vi "3_PatchCore_Report(Dataset).vi"(0 "NNFE PatchCore Paths":T1={"NNFE_Paths"={"CFG"=path "D:/PatchCore/__24_12_11__22_07_40/wrn_50_2_timm_NNFE__24_12_11__22_07_40.cfg", "BIN"=path "D:/PatchCore/__24_12_11__22_07_40/wrn_50_2_timm_NNFE__24_12_11__22_07_40.bin"}, "PatchCore_Paths"={"CFG"=path "D:/PatchCore/__24_12_11__22_07_40/wrn_50_2_timm_Patchcore__24_12_11__22_07_40.cfg", "BIN"=path "D:/PatchCore/__24_12_11__22_07_40/wrn_50_2_timm_MemBank__PS3_RP296_SR0.1_Size16.4k__24_12_11__22_07_40.bin"}}, 1 "NNFE_Custom_CFG":T11={"Input3D_Custom_Dims"={"C"=3, "H"=224, "W"=224}, "mBatch"=1}, 2 "Feature_Scorer_Params":T6={"Nearest_Neihbours"=1, "Calculate Anomaly Map"=TRUE, "Gaussian_Blur"={"Kernel_Size"=33, "sigma"=4.0}}, 3 "Report_Image_Dims":cluster{"X Resolution":i32, "Y Resolution":i32}={"X Resolution"=224, "Y Resolution"=224}, 7 "Eval_Stats_File_Path":path=path "D:/PatchCore/__24_12_11__22_07_40/PatchCore_Eval_Stats__24_12_11__22_13_40.cfg", 11 "Device_Config.":T3={"Device"=enum."GPU", "GPU Id"=0}, 12 "Image_Dataset_Folder_Path":path=path "D:/MVTec/bottle/test", 13 "Ground_Truth_Folder_Path":path=path "D:/MVTec/bottle/ground_truth", 14 "Dest. Path":path=path "D:/MVTec_Report/bottle") -> (6 "dt_Predict":dbl=0.010424548192794788 format="%#_4p")   [LabVIEW 2020]
uses:
  PatchCore_AddOn/API/Controls/NNPC_Init_Custom_NN_CFG.ctl
  <vilib>/Ngene/Deep Learning Toolkit/Toolkit/NN_Data/API/NN_Dims(C,H,W).ctl
  PatchCore_AddOn/API/Controls/Heatmap_Config.ctl
  PatchCore_AddOn/API/Controls/ColorMap.ctl
  PatchCore_AddOn/API/Controls/MinMax.ctl
  PatchCore_AddOn/API/Controls/Feature_Scorer_Params.ctl
  PatchCore_AddOn/API/Controls/Gaussian_Blur.ctl
  PatchCore_AddOn/API/Controls/NNPC_Device.ctl
  <vilib>/Ngene/Deep Learning Toolkit/Toolkit/NN_Network/Controls/NN_Device.ctl
  PatchCore_AddOn/API/Controls/NNPC_Trained_Model_Paths.ctl
  PatchCore_AddOn/API/Controls/NN_Paths.ctl
  subVIs/Dataset_Reader/Controls/ImRead_PreProcessing_Options.ctl
  PatchCore_AddOn/Low_Level/Controls/Normalization_Type.ctl
  <vilib>/Analysis/baseanly.llb/Mean (DBL).vi
  PatchCore_AddOn/API/NNPC_Predict/NNPC_Predict(Single).vi
  PatchCore_AddOn/PatchCore_AddOn.lvlib
  <vilib>/Analysis/NI_AALBase.lvlib
  <vilib>/Ngene/Deep Learning Toolkit/Toolkit/Deep_Learning_Toolkit_by_Ngene.lvlib
panel:
  out "Anomaly Detection Results":T5(plugin-control)
  out "Actual_Pixel_Threshold":sgl=25.5661
  out "Total":i32=83
  out "Progress":i32=82
  in  "Heatmap_Config":T8={"ColorMap_Type"=enum."Jet", "Alpha"=0.4, "Heatmap Range"={"Min"=-1.0, "Max"=-1.0}} {"Heatmap Range"."Min" format="%#_5g"}
  out "dT_ImRead":dbl=0.022437069879479934 format="%#_4p"
  in  "Pixel_Thrshld(Custom)":sgl=-1.0 format="%_5g"
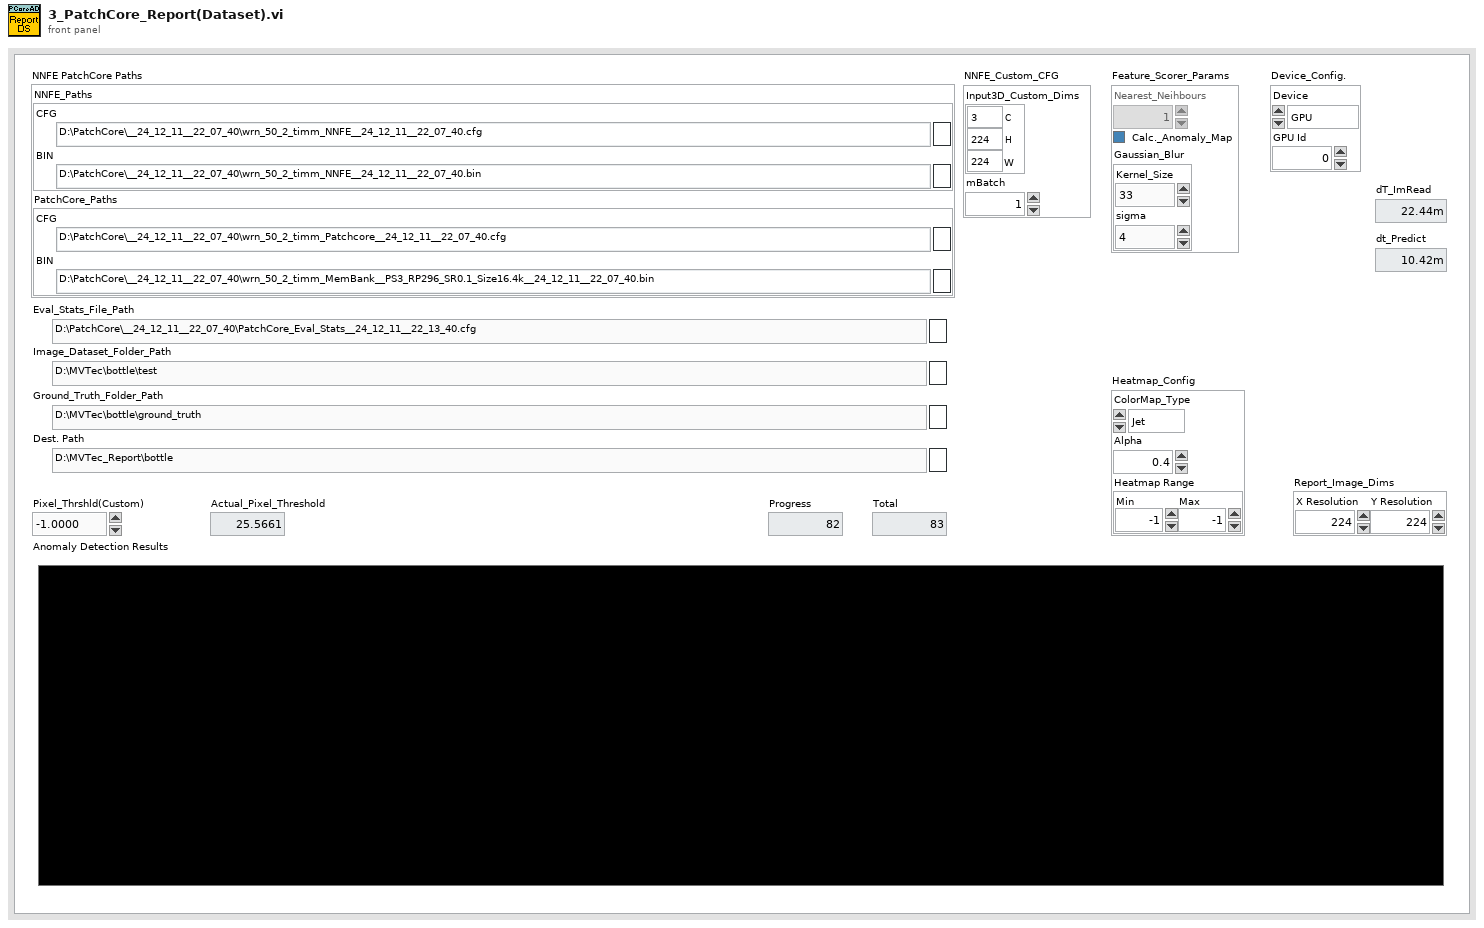
[diagram p1: front panel]
types:
  T1 = typedef "PatchCore_AddOn.lvlib/NNPC_Trained_Model_Paths.ctl" = cluster{"NNFE_Paths":T2, "PatchCore_Paths":T2}
  T2 = typedef "PatchCore_AddOn.lvlib/NN_Paths.ctl" = cluster{"CFG":path, "BIN":path}
  T3 = typedef "PatchCore_AddOn.lvlib/NNPC_Device.ctl" = cluster{"Device":T4, "GPU Id":i32}
  T4 = typedef "Deep_Learning_Toolkit_by_Ngene.lvlib/NN_Device.ctl" = enum16{"CPU", "GPU"}
  T5 = typedef "IMAQ Image.ctl" = refnum<image>
  T6 = typedef "PatchCore_AddOn.lvlib/Feature_Scorer_Params.ctl" = cluster{"Nearest_Neihbours":i32, "Calculate Anomaly Map":bool, "Gaussian_Blur":T7}
  T7 = typedef "PatchCore_AddOn.lvlib/Gaussian_Blur.ctl" = cluster{"Kernel_Size":i32, "sigma":sgl}
  T8 = typedef "PatchCore_AddOn.lvlib/Heatmap_Config.ctl" = cluster{"ColorMap_Type":T9, "Alpha":sgl, "Heatmap Range":T10}
  T9 = typedef "PatchCore_AddOn.lvlib/ColorMap.ctl" = enum16{"Jet", "Perula", "Inferno", "Plasma", "Viridis"}
  T10 = typedef "PatchCore_AddOn.lvlib/MinMax.ctl" = cluster{"Min":sgl, "Max":sgl}
  T11 = typedef "PatchCore_AddOn.lvlib/NNPC_Init_Custom_NN_CFG.ctl" = cluster{"Input3D_Custom_Dims":T12, "mBatch":i32}
  T12 = typedef "Deep_Learning_Toolkit_by_Ngene.lvlib/NN_Dims(C,H,W).ctl" = cluster{"C":i32, "H":i32, "W":i32}
  T13 = typedef "PatchCore_AddOn.lvlib/NNPC_Instance.ctl" = cluster{"Dataset_Stats":T14, "NN":T16, "Device_Config.":T3, "PatchCore_Init_CFG":T31, "Coreset Params":T33, "MemBank_Data":T35}
  T14 = typedef "PatchCore_AddOn.lvlib/NNPC_DS_Stats.ctl" = cluster{"means":T15, "vars":T15, "DS_Size":i32}
  T15 = typedef "PatchCore_AddOn.lvlib/Image_Stats_RGB.ctl" = cluster{"R":sgl, "G":sgl, "B":sgl}
  T16 = typedef "Deep_Learning_Toolkit_by_Ngene.lvlib/NN.ctl" = cluster{"Name":string, "No of Layers":i32, "mBatch":i32, "Layers":T17[], "Dimty":T18, "Dims_In":T12, "Dims_Out":T12, "Working_Dir":path, "Train?":bool, "Train_Params":T19, "LR_Update_Policy":T22, "Session Data":T24, "Ground_truth":T25, "NNg_hdls":T26, "NN_Device":T4, "GPU Id":i32, "Labels":string[], "Receptive Field":T27[], "Loss_Type":T28, "Loss_Cfg_Prms":variant, "NNG_WS":T29}
  T17 = typedef "Deep_Learning_Toolkit_by_Ngene.lvlib/NN_Layer_ref.ctl" = refnum<data-value>
  T18 = typedef "Deep_Learning_Toolkit_by_Ngene.lvlib/NN_In_Out_Dim-ty.ctl" = enum8{"In1D_Out1D", "In3D_Out1D", "In3D_Out3D", "In3D_OutBBox"}
  T19 = typedef "Deep_Learning_Toolkit_by_Ngene.lvlib/NN_Train_Params.ctl" = cluster{"Optimizer":T20, "Beta_1":sgl, "Beta_2":sgl, "Weight Decay(L1)":sgl, "Weight Decay(L2)":sgl, "Data_Sampling":T21}
  T20 = typedef "Deep_Learning_Toolkit_by_Ngene.lvlib/NN_Train_Optimizer.ctl" = enum16{"SGD", "Adam", "Adagrad", "Adadelta", "RMSProp", "Nesterov"}
  T21 = typedef "Deep_Learning_Toolkit_by_Ngene.lvlib/NN_Train_Data_Sampling.ctl" = enum16{"Random", "Sequential"}
  T22 = typedef "Deep_Learning_Toolkit_by_Ngene.lvlib/NN_LR_Policy_Cfg.ctl" = cluster{"Policy_Type":T23, "LR0":dbl, "k":sgl, "WarmUp_Policy":enum16{"Step", "Ramp"}, "WarmUp_Iter":i32, "WarmUp_Ratio":sgl}
  T23 = typedef "Deep_Learning_Toolkit_by_Ngene.lvlib/NN_LR_Policy_Type.ctl" = enum16{"Manual", "Step", "Exp", "1/t"}
  T24 = typedef "Deep_Learning_Toolkit_by_Ngene.lvlib/NN_Train_Session_Data.ctl" = cluster{"Epochs":sgl, "Tot_Iter":i32, "LR":sgl, "LR_iter":i32}
  T25 = typedef "Deep_Learning_Toolkit_by_Ngene.lvlib/NN_Ground_truth.ctl" = cluster{"Y":variant}
  T26 = typedef "Deep_Learning_Toolkit_by_Ngene.lvlib/nng_cuda_handles.ctl" = cluster{"cudnn":u64, "cublas":u64, "stream":u64, "curand":u64}
  T27 = typedef "Deep_Learning_Toolkit_by_Ngene.lvlib/NN_Dims(V,H).ctl" = cluster{"V":i32, "H":i32}
  T28 = typedef "Deep_Learning_Toolkit_by_Ngene.lvlib/NN_Loss_Type.ctl" = enum16{"None", "MSE", "CrossEntropy", "YOLO_v2", "YOLO_v4"}
  T29 = typedef "Deep_Learning_Toolkit_by_Ngene.lvlib/NNG_WS.ctl" = cluster{"NNG_WS_Mem":T30, "Max_WS_Size":i64}
  T30 = typedef "Deep_Learning_Toolkit_by_Ngene.lvlib/NNg_WS_Mem_DVR.ctl" = refnum<data-value>
  T31 = typedef "PatchCore_AddOn.lvlib/NNPC_Init_CFG.ctl" = cluster{"BackBone":T32, "Out_Layers_Names":string[], "Patch_Size":u32}
  T32 = typedef "PatchCore_AddOn.lvlib/NNPC_BackBone_Selector.ctl" = enum16{"WRN_50_2_L2L3"}
  T33 = typedef "PatchCore_AddOn.lvlib/NNPC_Coreset_Params.ctl" = cluster{"Name":string, "Sampling_Ratio":sgl, "Startd_idx":i32, "Random_Proj?":bool, "Rnd. Proj. Params":T34}
  T34 = typedef "PatchCore_AddOn.lvlib/NNPC_Random_Projection_CFG.ctl" = cluster{"Proj._Dim.":i32, "Epsilon":sgl, "Seed":i32}
  T35 = typedef "PatchCore_AddOn.lvlib/MemBank_and_Norm_Variants.ctl" = cluster{"MemBank":variant, "MemBank Norm":variant}
  T36 = typedef "PatchCore_AddOn.lvlib/Eval_Results.ctl" = cluster{"Scores(Good)":T10, "Scores(Bad)":T10, "F1_Max":sgl, "Thrshld(F1_Max)":sgl, "IoU_Max":sgl, "Thrshld(IoU_Max)":sgl, "AUROC":sgl, "Prec.(F1_Max)":sgl, "Recall(F1_Max)":sgl, "FPR(F1_Max)":sgl, "FNR(F1_Max)":sgl}
  T37 = enum16{"open", "replace", "create", "open or create", "replace or create", "replace or create with confirmation"}
  T38 = typedef "ImRead_PreProcessing_Options.ctl" = cluster{"Image Type":T39, "Normalization Type":T40, "Interpolation Type":u32}
  T39 = typedef "Image Type" = u32
  T40 = typedef "PatchCore_AddOn.lvlib/Normalization_Type.ctl" = enum16{"Standardize(DS_Stats)", "Standardize(Image_Stats)"}
  T41 = typedef "PatchCore_AddOn.lvlib/Anomaly_Detection_Results_Imgs.ctl" = cluster{"Image":T5, "Ground Truth":T5, "Predicted Heat Map":T5, "Predicted Mask":T5, "Segmentation":T5}
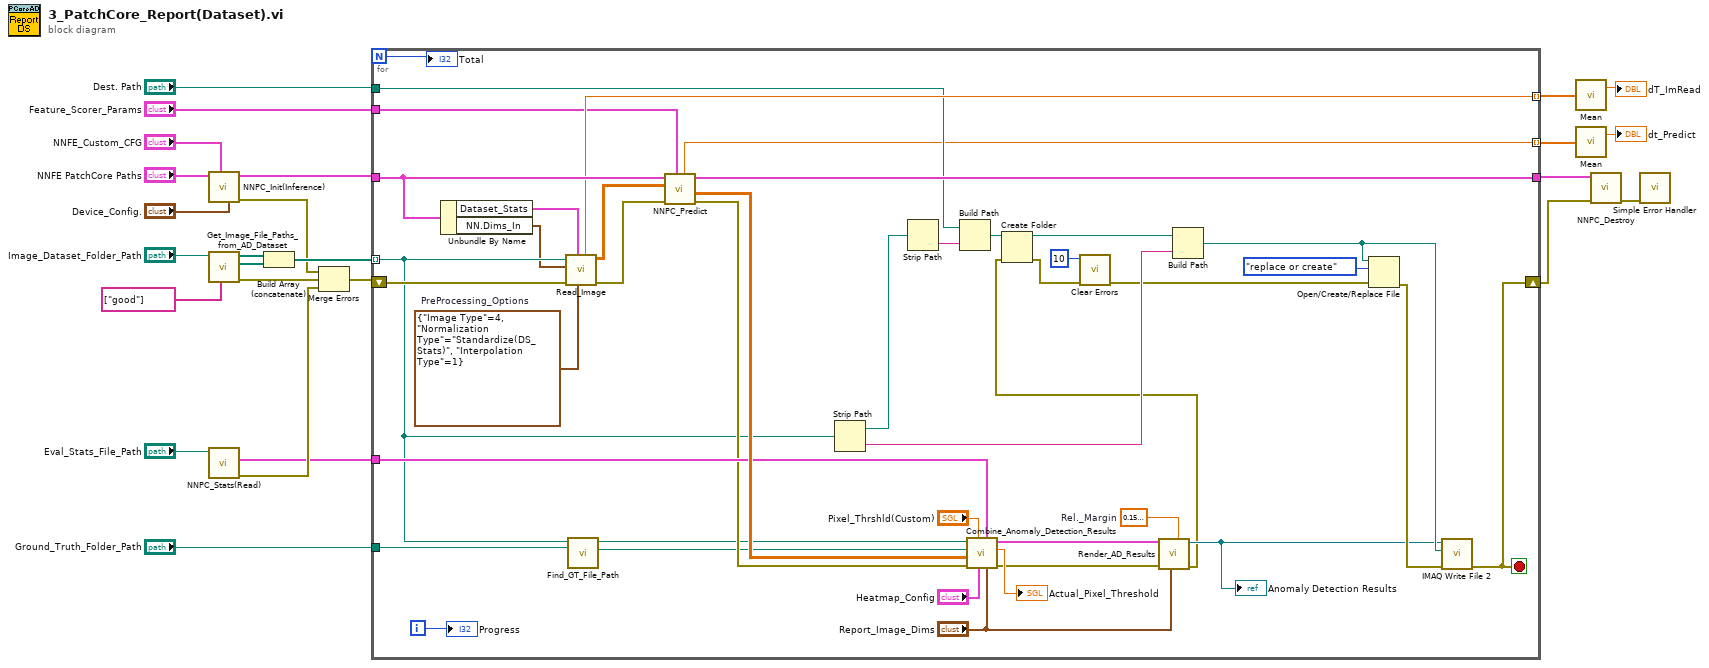
[diagram p0: block diagram]
diagram:
  n1 = call "NNPC_Init(Inference).vi"("Device_Config."="Device_Config.", "NNFE_Custom_CFG"="NNFE_Custom_CFG", "NNFE PatchCore Paths"="NNFE PatchCore Paths") -> ("error out"=w5:errorcluster, "PCore_Instance out"=w22:T13)  [unwired: 7 in]
  n2 = call "Get_Image_File_Paths_from_AD_Dataset.vi"("Good Folder Names"=string[] ["good"] ("Good Folder Name"), "Dataset Folder"="Image_Dataset_Folder_Path") -> ("error out"=w20:errorcluster, "Bad Dataset Files"=w12:path[], "Good Dataset Files"=w13:path[])  [unwired: 7 in]
  n3 = call "NNPC_Stats(Read).vi"("CFG file path"="Eval_Stats_File_Path") -> ("error out"=w19:errorcluster, "Pixel Results"=w10:T36)  [unwired: 8 in, 1 out]
  n4 = Build Array (concatenate)(w13, w12) -> (w11:path[])
  n5 = Merge Errors(w5, w20, w19) -> (w4:errorcluster)
  n6 = for {
    N -> [w42]
    shift-right: [w52] -> w24
    shift-left: w4 -> [w67]
    tunnel: w11 -> [w35] mode=indexing
    tunnel: w22 -> [w63]
    tunnel: [w66] -> w7
    tunnel: w10 -> [w58]
    tunnel: [w56] -> w16 mode=indexing
    tunnel: [w37] -> w15 mode=indexing
    tunnel: "Dest. Path" -> [w53]
    tunnel: "Ground_Truth_Folder_Path" -> [w40]
    tunnel: "Feature_Scorer_Params" -> [w31]
    i -> [w43]
    stop <- w52 stop-if-true
    w27 = T38 {"Image Type"=4, "Normalization Type"=enum."Standardize(DS_Stats)", "Interpolation Type"=1}  # PreProcessing_Options
    w60 = sgl 0.15  # Rel._Margin
    n7 = Unbundle By Name(w63) -> ("Dataset_Stats"=w29:T14, "NN.Dims_In"=w28:T12)
    n8 = call "Read_Image.vi"("PreProcessing_Options"=w27, "Dataset_Stats"=w29, "error in"=w67, "Target_Dims"=w28, "Img Path"=w35) -> ("error out"=w62:errorcluster, "Image Out"=w30:sgl[][][], "dT_Img_Read"=w56:dbl)  [unwired: 4 in]
    n9 = call "Find_GT_File_Path.vi"("GT Mask Folder Path"=w40, "Image File Path"=w35) -> ("GT File Path"=w38:path, "Image File Path out"=w39:path)  [unwired: 8 in]
    n10 = call-poly "NNPC_Predict.vi"("Feature Scorer Params"=w31, "error in"=w62, "Image in"=w30, "PCore_Instance in"=w63) -> ("error out"=w47:errorcluster, "anomaly map"=w65:sgl[][], "PCore_Instance out"=w66:T13, "dT_Predict"=w37:dbl)  [unwired: 3 in, 1 out]
    n11 = Strip Path(path=w35) -> (stripped path=w55:path, name=w54:string)
    n12 = Strip Path(path=w55) -> (name=w33:string)  [unwired: 1 out]
    n13 = Build Path(base path=w53, name or relative path=w33) -> (appended path=w34:path)
    n14 = call "Combine_Anomaly_Detection_Results.vi"("Infrnc Dims"="Report_Image_Dims", "Pixel Results"=w58, "Heatmap Config"="Heatmap_Config", "Pixel Anomaly Thrshld"="Pixel_Thrshld(Custom)", "error in"=w47, "Anomaly Map"=w65, "Gt File Path"=w38, "Img File Path"=w39) -> ("error out"=w26:errorcluster, "Actual Pixel Threshold"=→"Actual_Pixel_Threshold":sgl, "Anomaly Detection Rresults"=w64:T41)  [unwired: 1 in]
    n15 = call "Render_AD_Results.vi"("Rel._Margin"=w60, "Image_Dims"="Report_Image_Dims", "error in"=w26, "Anomaly Detection Rresults"=w64) -> ("error out"=w32:errorcluster, "Anomaly Detection Results"=w36:T5)  [unwired: 6 in]
    "Anomaly Detection Results" <- w36
    n16 = Create Folder(path (use dialog)=w34, error in=w32) -> (created path=w48:path, error out=w46:errorcluster)  [unwired: 1 in, 1 out]
    n17 = call <vilib>:"Clear Errors.vi"("error in (no error)"=w46, "specific error code to clear (0: all)"=10) -> ("error out"=w45:errorcluster)  [unwired: 4 in, 1 out]
    n18 = Build Path(base path=w48, name or relative path=w54) -> (appended path=w51:path)
    n19 = Open/Create/Replace File(file path (use dialog)=w51, error in=w45, operation (0:open)=T37."replace or create") -> (error out=w50:errorcluster)  [unwired: 3 in, 2 out]
    n20 = call-poly "IMAQ Write File 2"("error in (no error)"=w50, "File Path"=w51, "Image"=w36) -> ("error out"=w52:errorcluster)  [unwired: 7 in, 1 out]
    "Progress" <- w43
    "Total" <- w42
  }
  n21 = call-poly <vilib>:"Mean.vi"("X"=w16) -> ("mean"=→"dT_ImRead":dbl)  [unwired: 1 out]
  n22 = call-poly <vilib>:"Mean.vi"("X"=w15) -> ("mean"=→"dt_Predict":dbl)  [unwired: 1 out]
  n23 = call "NNPC_Destroy.vi"("error in"=w24, "PCore_Instance in"=w7) -> ("error out"=w23:errorcluster)  [unwired: 9 in]
  n24 = call <vilib>:"Simple Error Handler.vi"("error in (no error)"=w23) -> ()  [unwired: 4 in, 5 out]
